vi "from string array.vi"(8 "error in (no error)":errorcluster, 9 "String Array":string[][](array[string]), 10 "version":string, 11 "Sequencer Module configuration in":refnum<class "Sequencer Module configuration.lvclass">) -> (0 "error out":errorcluster, 3 "Sequencer Module configuration out":refnum<class "Sequencer Module configuration.lvclass">)   [LabVIEW 2015, in "Sequencer Module configuration.lvclass"]
uses:
  Sequencer Module configuration.lvclass
  <vilib>/NI/Tag Bus/tag/Data Type.ctl
  Line.ctl
  <vilib>/NI/Tag Bus Module Framework/channel/TBM channel.lvclass
  permissions.ctl
  Sequencer Module configuration.lvclass/Sequencer Module configuration.ctl
  Write Lines.vi
  Get Line Name.vi
  <vilib>/NI/Tag Bus Module Framework/module configuration/FindDuplicate.vi
  <vilib>/Utility/error.llb/Error Cluster From Error Code.vi
  <vilib>/NI/Tag Bus/tag/tag descriptor.lvclass
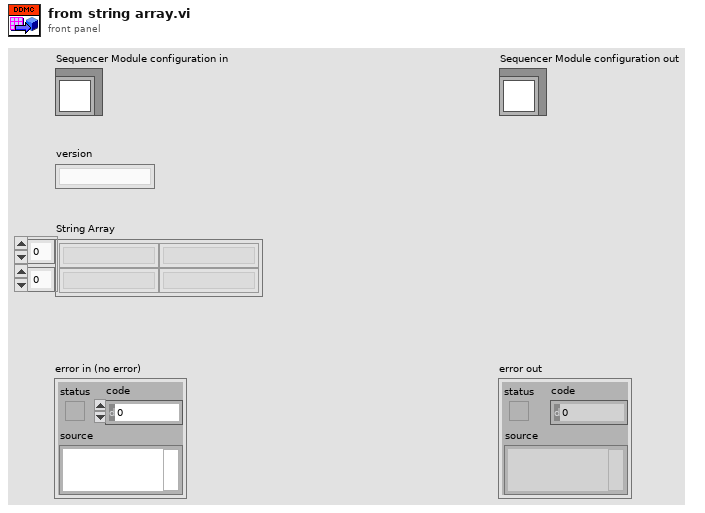
[diagram p1: front panel]
types:
  T1 = typedef "Sequencer Module configuration.lvclass/permissions.ctl" = enum32{"Read from HW", "Write to HW"}
  T2 = typedef "Sequencer Module configuration.lvclass/Line.ctl" = cluster{"channel":refnum<class "TBM channel.lvclass">}
  T3 = typedef "tag bus.lvlib/tag descriptor.lvclass/Data Type.ctl" = enum16{"Double", "Single", "I64", "I32", "I16", "I8", "U64", "U32", "U16", "U8", "Boolean", "String", "Array of Double", "Array of Single", "Array of I64", "Array of I32", "Array of I16", "Array of I8", "Array of U64", "Array of U32", "Array of U16", "Array of U8", "Array of Boolean", "Array of String"}
  T4 = typedef "TBM channel.lvclass/channel classification.ctl" = enum16{"input data", "output data", "processing parameter", "processing result"}
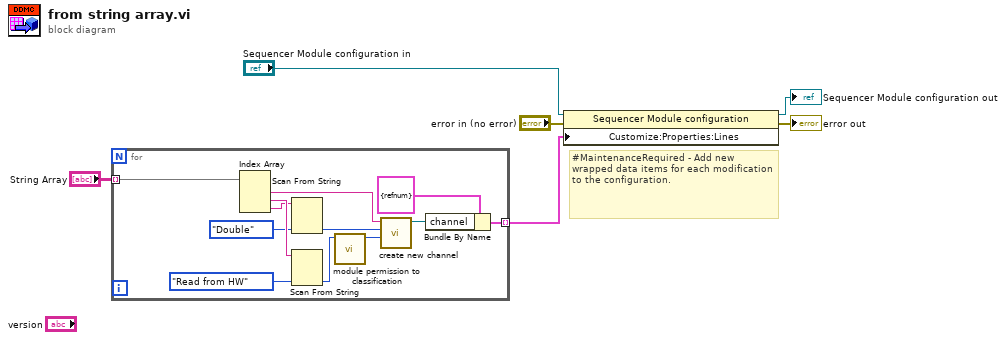
[diagram p0: block diagram]
diagram:
  # "#MaintenanceRequired - Add new wrapped data items for each modification to the configuration."
  n1 = for {
    tunnel: "String Array" -> [w18] mode=indexing
    tunnel: [w11] -> w1 mode=indexing
    n2 = Index Array(array=w18) -> (element #1=w17:string, element #2=w16:string, element #3=w15:string)  [unwired: 3 in]
    n3 = Scan From String(input string=w15, default 1=Data_Type."Double" ("data type")) -> (output 1=w13:T3)  [unwired: 3 in, 3 out]
    n4 = Scan From String(input string=w16, default 1=permissions."Read from HW" ("view direction")) -> (output 1=w8:T1)  [unwired: 3 in, 3 out]
    n5 = call "module permission to classification.vi"("display permissions"=w8) -> ("channel classification"=w7:T4)  [unwired: 10 in]
    n6 = call <vilib>:"create new channel.vi"("channel classification"=w7, "data type"=w13, "channel name"=w17) -> ("channel"=w12:refnum<class "TBM channel.lvclass">)  [unwired: 8 in]
    n7 = Bundle By Name(cluster=T2 {"channel"=refnum} ("Line"), "channel"=w12) -> (w11:T2)
  }
  n8 = property class="Sequencer Module configuration"(reference="Sequencer Module configuration in", error in="error in (no error)", "Customize:Properties:Lines"=w1) -> (reference out=→"Sequencer Module configuration out":refnum<class "Sequencer Module configuration.lvclass">, error out=→"error out":errorcluster)
